vi "n4_betas.vi"(4 "Time":dbl[](array[numeric]), 5 "Tamaño Sn":i32[](array[numeric]), 6 "Analysis":u8, 8 "m":dbl, 9 "P":dbl, 10 "Segmentation A":dbl[](array[numeric]), 11 "Segmentation B":dbl[](array[numeric])) -> (0 "bB":dbl, 1 "X2_tau":dbl[][](array[numeric]), 2 "X2_i":dbl[][](array[numeric]), 3 "bA":dbl)   [LabVIEW 2015]
uses:
  <vilib>/Analysis/baseanly.llb/Mean (DBL).vi
  <vilib>/Analysis/NI_AALBase.lvlib
  <vilib>/Analysis/NI_AALPro.lvlib
panel:
  out "bB_anterior":dbl
  out "bA_anterior":dbl
  out "output array 4":dbl[](array[numeric])
  out "MA 3":dbl
  out "MB 2":dbl
  out "MA 2":dbl
  out "output array 2":dbl[](array[numeric])
  out "MB":dbl
  out "MA":dbl
  out "output array":dbl[](array[numeric])
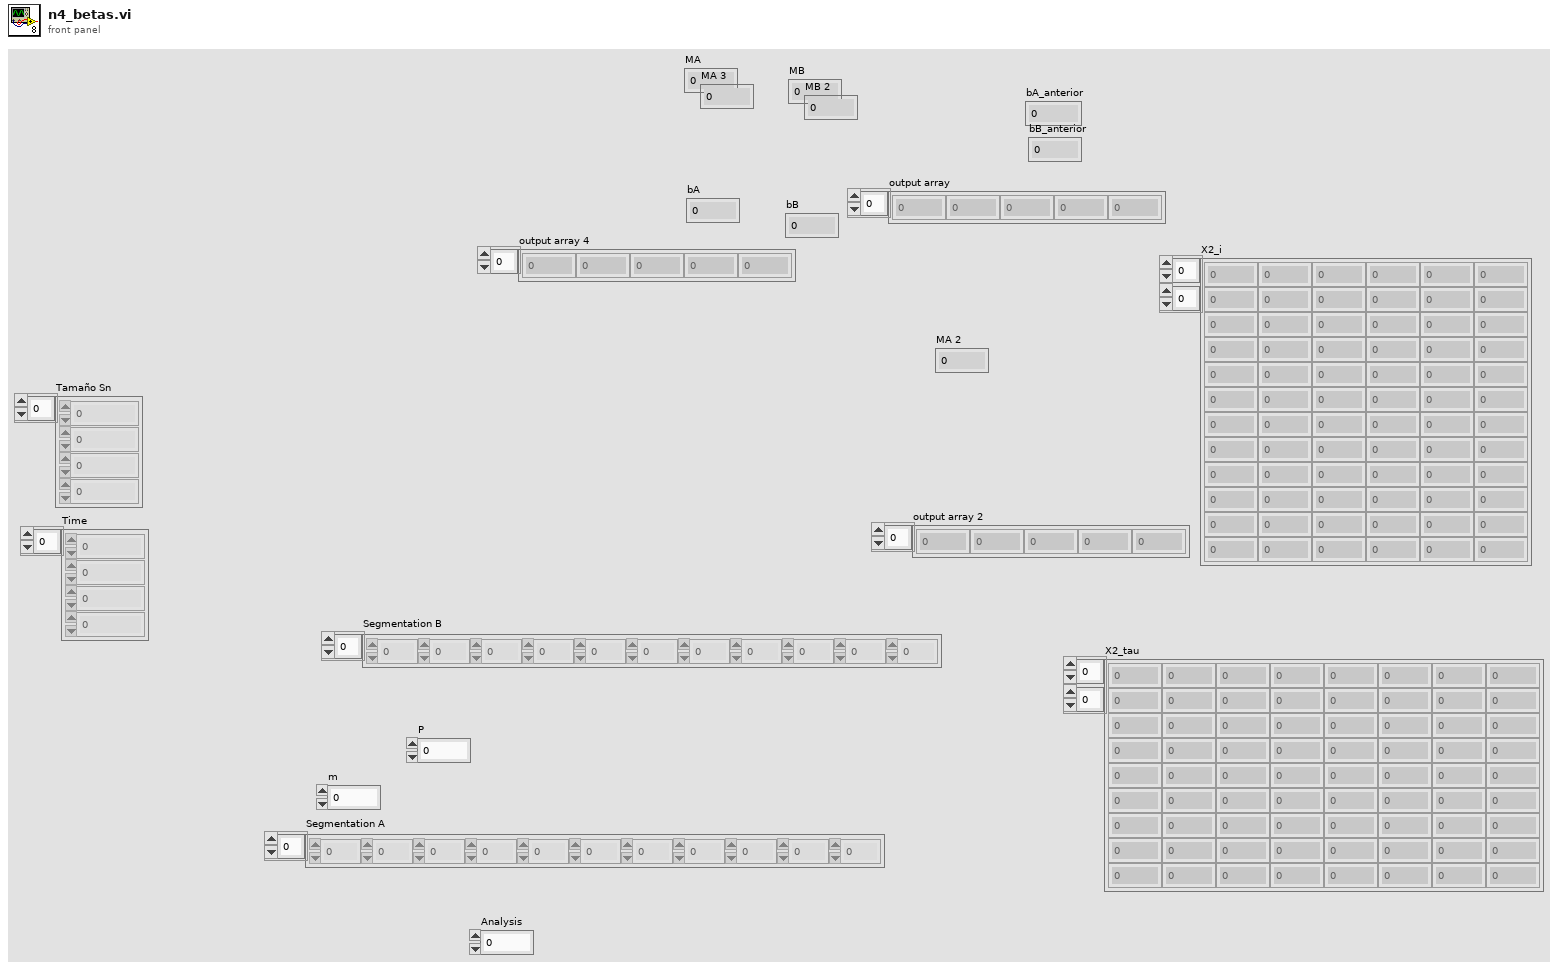
[diagram p1: front panel]
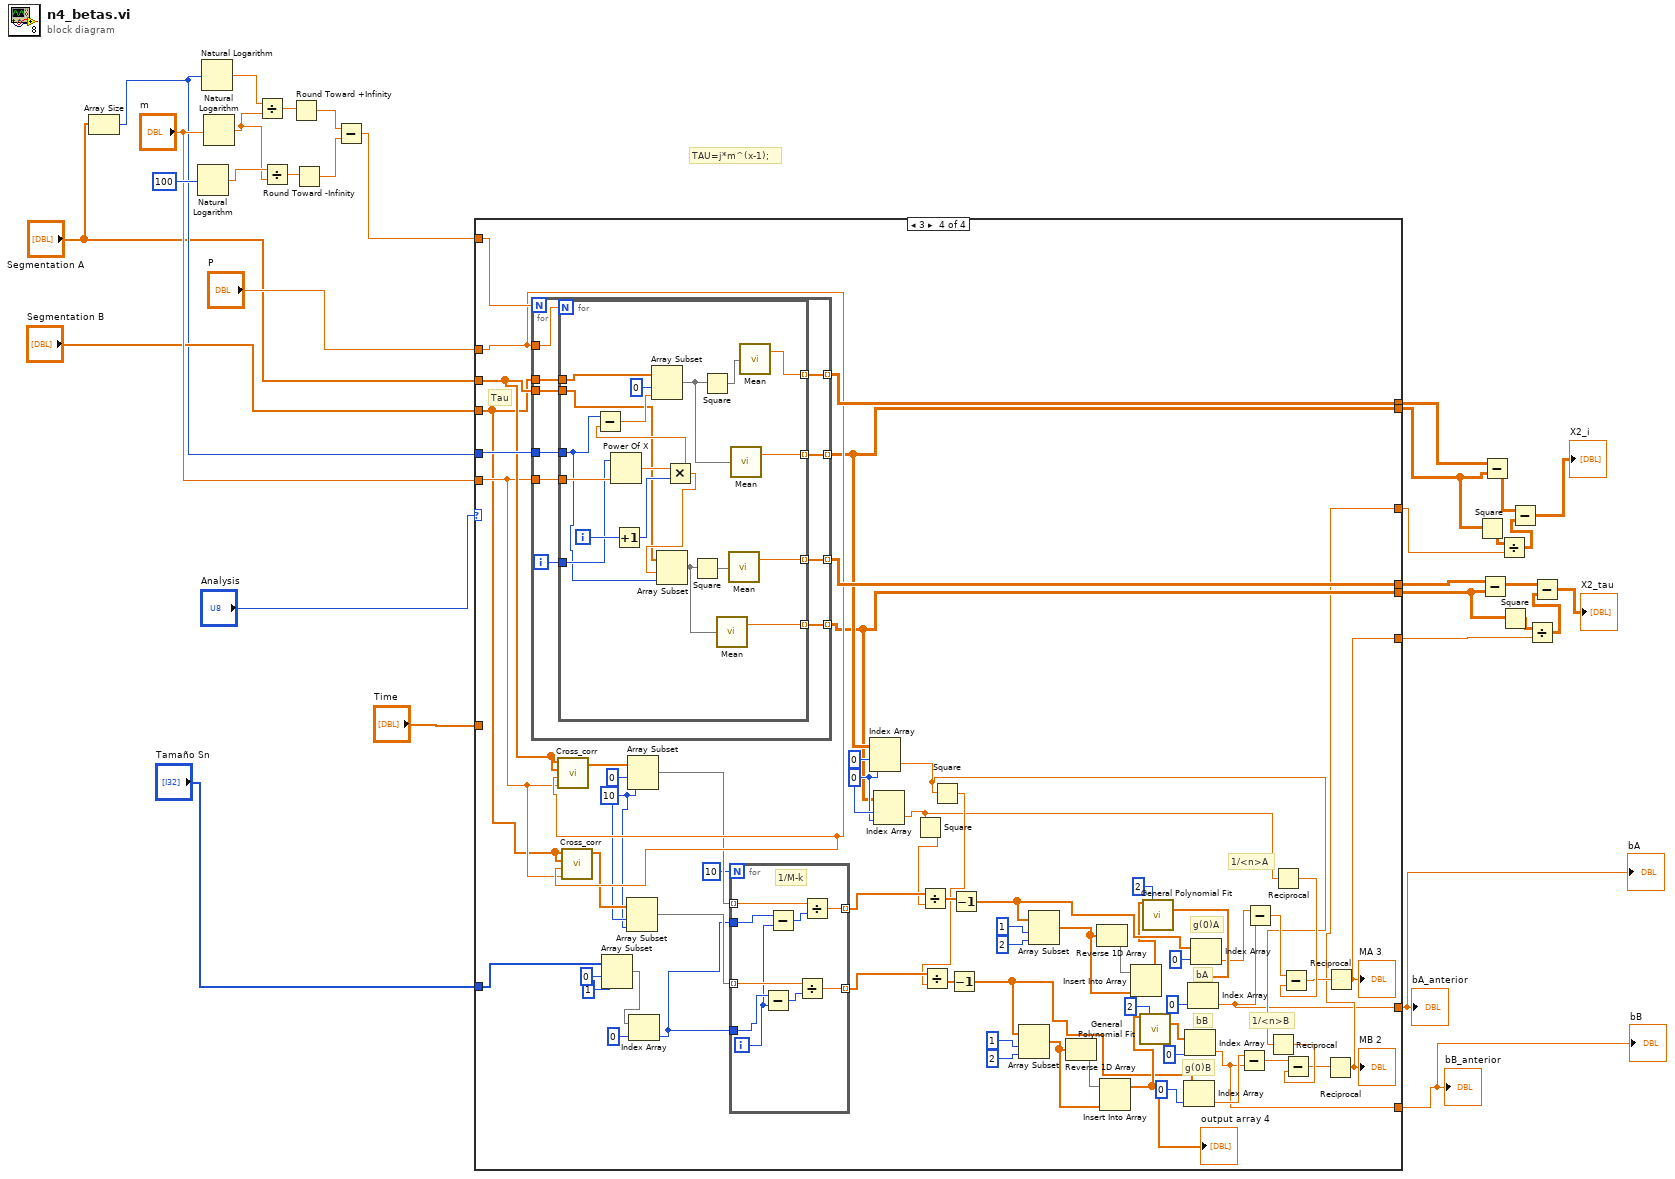
[diagram p0: block diagram]
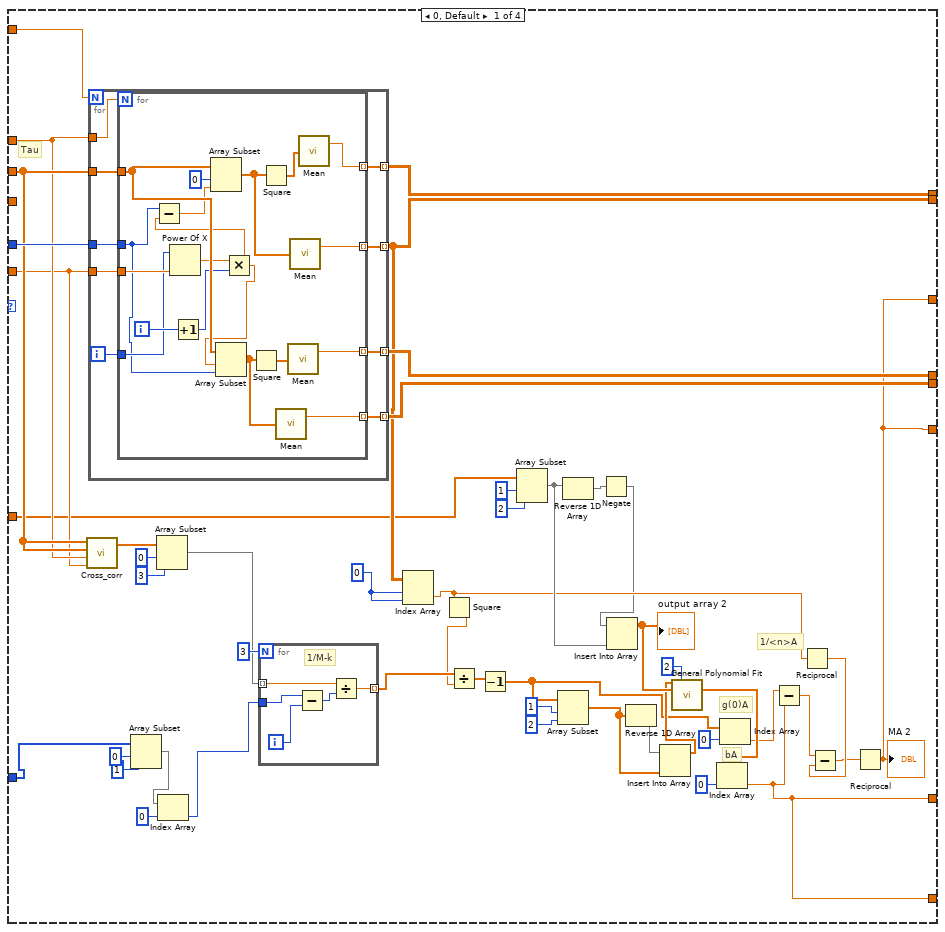
[diagram p2: hidden frame]
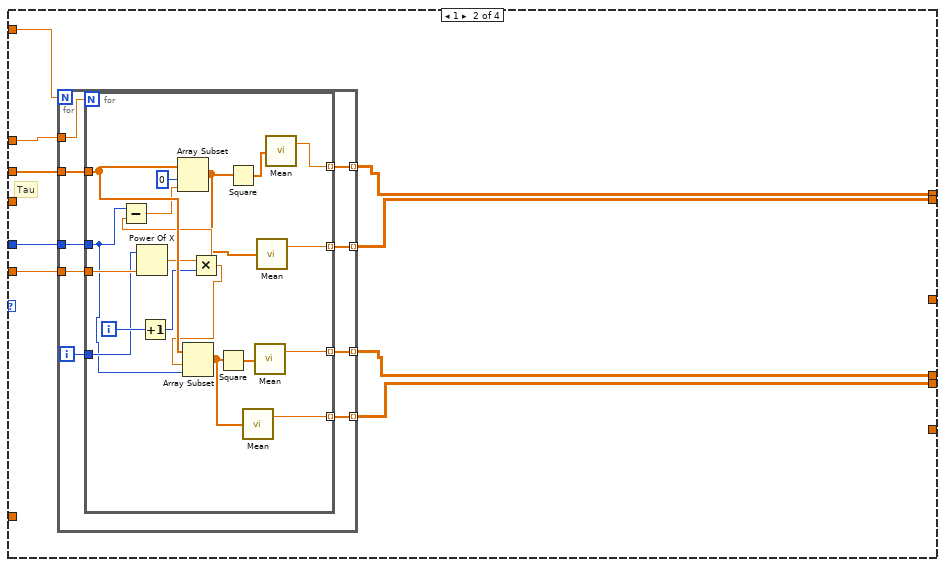
[diagram p3: hidden frame]
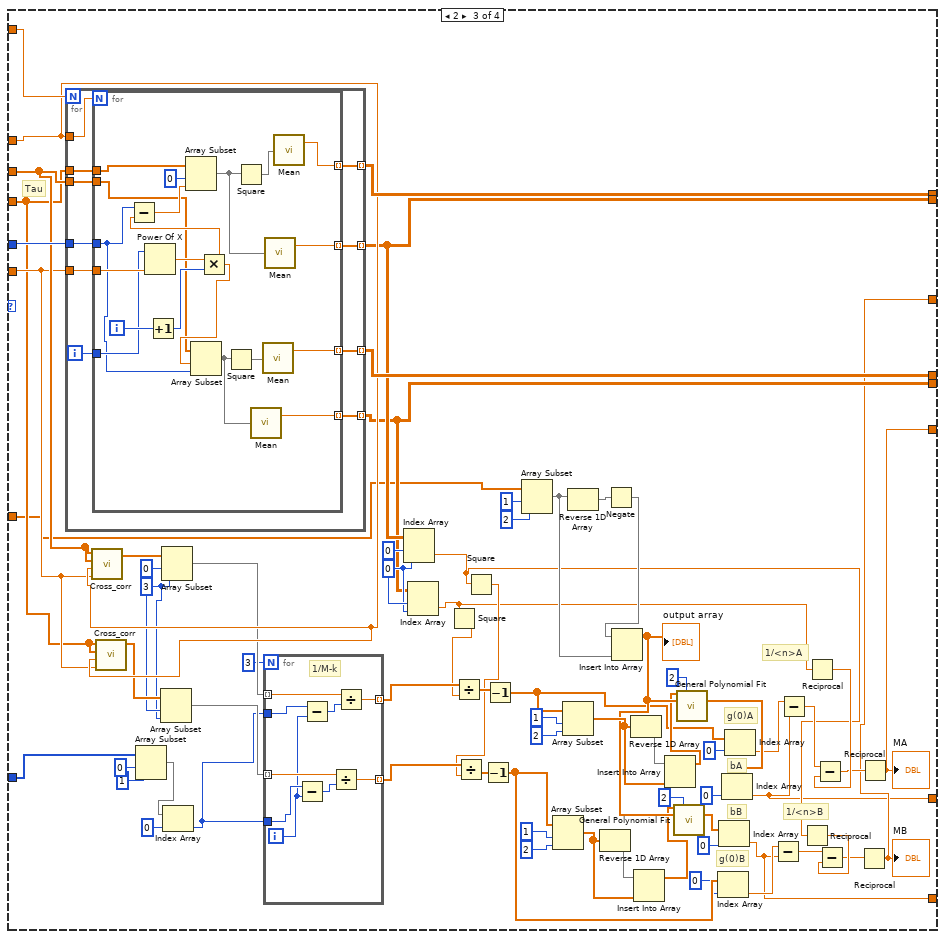
[diagram p4: hidden frame]
diagram:
  # "TAU=j*m^(x-1);"
  n1 = Array Size(array="Segmentation A") -> (size(s)=w18:i32)
  n2 = Natural Logarithm(1:100) -> (0:w30:dbl)
  n3 = Natural Logarithm(1:w18) -> (0:w33:dbl)
  n4 = Natural Logarithm(1:"m") -> (0:w29:dbl)
  n5 = Divide(x=w33, y=w29) -> (x/y=w32:dbl)
  n6 = Divide(x=w30, y=w29) -> (x/y=w27:dbl)
  n7 = Round Toward +Infinity(x=w32) -> (ceil(x): smallest int >= x=w28:dbl)
  n8 = Round Toward -Infinity(1:w27) -> (0:w26:dbl)
  n9 = Subtract(x=w28, y=w26) -> (x-y=w25:dbl)
  n10 = case shown="3" "Analysis" {
    tunnel: "Segmentation A" -> [w45 w122 w217 w320]
    tunnel: w18 -> [w77 w121 w220 w323]
    tunnel: w25 -> [w78 w120 w221 w324]
    tunnel: "m" -> [w43 w119 w215 w318]
    tunnel: "P" -> [w44 w118 w216 w319]
    tunnel: [w81 w117 w219 w322] -> w20
    tunnel: [w40 w116 w202 w305] -> w14
    tunnel: [w80 w115 w218 w321] -> w19
    tunnel: [w79 w114 w177 w288] -> w15
    tunnel: "Segmentation B" -> [_ _ w156 w269]
    tunnel: "Tamaño Sn" -> [w46 _ w208 w311]
    tunnel: [w39 _ w155 w268] -> w12
    tunnel: [w39 _ w154 w267] -> w7
    tunnel: "Time" -> [w35 _ w152 _]
    tunnel: [w34 _ w151 w265] -> w2
    tunnel: [w34 _ w150 w264] -> w1
    frame 0, Default {
      w41 = 0 ("index (col)")
      # "1/<n>A"
      # "bA"
      # "g(0)A"
      # "Tau"
      n11 = call "Cross_corr.vi"("m"=w43, "P"=w44, "input B"=w45, "input A"=w45) -> ("Acc"=w76:dbl[])  [unwired: 5 in, 2 out]
      n12 = for {
        N: w78 -> [_]
        tunnel: w44 -> [w95]
        tunnel: w45 -> [w94]
        tunnel: w77 -> [w93]
        tunnel: w43 -> [w92]
        tunnel: [w91] -> w81 mode=indexing
        tunnel: [w90] -> w40 mode=indexing
        tunnel: [w88] -> w80 mode=indexing
        tunnel: [w87] -> w79 mode=indexing
        i -> [w89]
        n13 = for {
          N: w95 -> [_]
          tunnel: w94 -> [w110]
          tunnel: w93 -> [w102]
          tunnel: w92 -> [w113]
          tunnel: w89 -> [w104]
          tunnel: [w112] -> w91 mode=indexing
          tunnel: [w111] -> w90 mode=indexing
          tunnel: [w108] -> w88 mode=indexing
          tunnel: [w107] -> w87 mode=indexing
          i -> [w106]
          n14 = Power Of X(1:w113, 2:w104) -> (0:w96:dbl)
          n15 = Increment(x=w106) -> (x+1=w105:i32)
          n16 = Multiply(x=w96, y=w105) -> (x*y=w103:dbl)
          n17 = Subtract(x=w102, y=w103) -> (x-y=w100:dbl)
          n18 = Array Subset(array=w110, index=0, length=w100) -> (w101:dbl[])
          n19 = Array Subset(array=w110, index=w103, length=w102) -> (w97:dbl[])
          n20 = Square(x=w97) -> (x^2=w109:dbl[])
          n21 = Square(x=w101) -> (x^2=w98:dbl[])
          n22 = call-poly <vilib>:"Mean.vi"("X"=w97) -> ("mean"=w107:dbl)  [unwired: 1 out]
          n23 = call-poly <vilib>:"Mean.vi"("X"=w109) -> ("mean"=w108:dbl)  [unwired: 1 out]
          n24 = call-poly <vilib>:"Mean.vi"("X"=w101) -> ("mean"=w111:dbl)  [unwired: 1 out]
          n25 = call-poly <vilib>:"Mean.vi"("X"=w98) -> ("mean"=w112:dbl)  [unwired: 1 out]
        }
      }
      n26 = Array Subset(array=w46, index=0, length=1) -> (w71:i32[])
      n27 = Array Subset(array=w76, index=0, length=3) -> (w37:dbl[])
      n28 = Index Array(array=w71, index=0) -> (element=w42:i32)
      n29 = for {
        N: 3 -> [_]
        tunnel: w37 -> [w85] mode=indexing
        tunnel: w42 -> [w84]
        tunnel: [w82] -> w69 mode=indexing
        i -> [w83]
        # "1/M-k"
        n30 = Subtract(x=w84, y=w83) -> (x-y=w86:i32)
        n31 = Divide(x=w85, y=w86) -> (x/y=w82:dbl)
      }
      n32 = Index Array(array=w40, index (row)=w41, index (col)=w41) -> (element=w50:dbl)
      n33 = Square(x=w50) -> (x^2=w56:dbl)
      n34 = Divide(x=w69, y=w56) -> (x/y=w68:dbl[])
      n35 = Decrement(x=w68) -> (x-1=w55:dbl[])
      n36 = Array Subset(array=w35, index=1, length=2) -> (w60:dbl[])
      n37 = Array Subset(array=w55, index=1, length=2) -> (w59:dbl[])
      n38 = Reverse 1D Array(array=w60) -> (reversed array=w65:dbl[])
      n39 = Negate(x=w65) -> (-x=w36:dbl[])
      n40 = Insert Into Array(array=w36, new element=w60) -> (w58:dbl[])  [unwired: 1 in]
      "output array 2" <- w58
      n41 = Reverse 1D Array(array=w59) -> (reversed array=w61:dbl[])
      n42 = Insert Into Array(array=w61, new element=w59) -> (w57:dbl[])  [unwired: 1 in]
      n43 = call <vilib>:"General Polynomial Fit.vi"("Y"=w57, "polynomial order"=2, "X"=w58) -> ("Polynomial Coefficients"=w53:dbl[])  [unwired: 9 in, 3 out]
      n44 = Index Array(array=w53, index=0) -> (element=w34:dbl)
      n45 = Index Array(array=w55, index=0) -> (element=w51:dbl)
      n46 = Subtract(x=w51, y=w34) -> (x-y=w49:dbl)
      n47 = Reciprocal(x=w50) -> (1/x=w48:dbl)
      n48 = Subtract(x=w49, y=w48) -> (x-y=w47:dbl)
      n49 = Reciprocal(x=w47) -> (1/x=w39:dbl)
      "MA 2" <- w39
    }
    frame 1 {
      # "Tau"
      n50 = for {
        N: w120 -> [_]
        tunnel: w118 -> [w131]
        tunnel: w122 -> [w130]
        tunnel: w121 -> [w129]
        tunnel: w119 -> [w128]
        tunnel: [w127] -> w117 mode=indexing
        tunnel: [w126] -> w116 mode=indexing
        tunnel: [w124] -> w115 mode=indexing
        tunnel: [w123] -> w114 mode=indexing
        i -> [w125]
        n51 = for {
          N: w131 -> [_]
          tunnel: w130 -> [w146]
          tunnel: w129 -> [w136]
          tunnel: w128 -> [w149]
          tunnel: w125 -> [w139]
          tunnel: [w148] -> w127 mode=indexing
          tunnel: [w147] -> w126 mode=indexing
          tunnel: [w144] -> w124 mode=indexing
          tunnel: [w142] -> w123 mode=indexing
          i -> [w141]
          n52 = Power Of X(1:w149, 2:w139) -> (0:w138:dbl)
          n53 = Increment(x=w141) -> (x+1=w140:i32)
          n54 = Multiply(x=w138, y=w140) -> (x*y=w137:dbl)
          n55 = Subtract(x=w136, y=w137) -> (x-y=w134:dbl)
          n56 = Array Subset(array=w146, index=0, length=w134) -> (w135:dbl[])
          n57 = Array Subset(array=w146, index=w137, length=w136) -> (w143:dbl[])
          n58 = Square(x=w143) -> (x^2=w145:dbl[])
          n59 = Square(x=w135) -> (x^2=w132:dbl[])
          n60 = call-poly <vilib>:"Mean.vi"("X"=w143) -> ("mean"=w142:dbl)  [unwired: 1 out]
          n61 = call-poly <vilib>:"Mean.vi"("X"=w145) -> ("mean"=w144:dbl)  [unwired: 1 out]
          n62 = call-poly <vilib>:"Mean.vi"("X"=w135) -> ("mean"=w147:dbl)  [unwired: 1 out]
          n63 = call-poly <vilib>:"Mean.vi"("X"=w132) -> ("mean"=w148:dbl)  [unwired: 1 out]
        }
      }
    }
    frame 2 {
      w200 = 0 ("index (col)")
      w201 = 0 ("index (row)")
      w153 = 3 ("length")
      w212 = 0 ("index")
      # "1/<n>B"
      # "1/<n>A"
      # "bB"
      # "bA"
      # "g(0)B"
      # "g(0)A"
      # "Tau"
      n64 = for {
        N: w221 -> [_]
        tunnel: w216 -> [w240]
        tunnel: w156 -> [w239]
        tunnel: w220 -> [w238]
        tunnel: w215 -> [w237]
        tunnel: [w236] -> w219 mode=indexing
        tunnel: [w235] -> w202 mode=indexing
        tunnel: [w233] -> w218 mode=indexing
        tunnel: [w232] -> w177 mode=indexing
        tunnel: w217 -> [w231]
        i -> [w234]
        n65 = for {
          N: w240 -> [_]
          tunnel: w239 -> [w242]
          tunnel: w238 -> [w247]
          tunnel: w237 -> [w259]
          tunnel: w234 -> [w250]
          tunnel: [w258] -> w236 mode=indexing
          tunnel: [w257] -> w235 mode=indexing
          tunnel: [w255] -> w233 mode=indexing
          tunnel: [w253] -> w232 mode=indexing
          tunnel: w231 -> [w241]
          i -> [w252]
          n66 = Power Of X(1:w259, 2:w250) -> (0:w249:dbl)
          n67 = Increment(x=w252) -> (x+1=w251:i32)
          n68 = Multiply(x=w249, y=w251) -> (x*y=w248:dbl)
          n69 = Subtract(x=w247, y=w248) -> (x-y=w245:dbl)
          n70 = Array Subset(array=w242, index=0, length=w245) -> (w246:dbl[])
          n71 = Array Subset(array=w241, index=w248, length=w247) -> (w254:dbl[])
          n72 = Square(x=w254) -> (x^2=w256:dbl[])
          n73 = Square(x=w246) -> (x^2=w243:dbl[])
          n74 = call-poly <vilib>:"Mean.vi"("X"=w254) -> ("mean"=w253:dbl)  [unwired: 1 out]
          n75 = call-poly <vilib>:"Mean.vi"("X"=w256) -> ("mean"=w255:dbl)  [unwired: 1 out]
          n76 = call-poly <vilib>:"Mean.vi"("X"=w246) -> ("mean"=w257:dbl)  [unwired: 1 out]
          n77 = call-poly <vilib>:"Mean.vi"("X"=w243) -> ("mean"=w258:dbl)  [unwired: 1 out]
        }
      }
      n78 = call "Cross_corr.vi"("m"=w215, "P"=w216, "input B"=w217, "input A"=w217) -> ("Acc"=w214:dbl[])  [unwired: 5 in, 2 out]
      n79 = call "Cross_corr.vi"("m"=w215, "P"=w216, "input B"=w156, "input A"=w156) -> ("Acc"=w213:dbl[])  [unwired: 5 in, 2 out]
      n80 = Array Subset(array=w208, index=0, length=1) -> (w205:i32[])
      n81 = Array Subset(array=w213, index=w212, length=w153) -> (w210:dbl[])
      n82 = Array Subset(array=w214, index=w212, length=w153) -> (w211:dbl[])
      n83 = Index Array(array=w205, index=0) -> (element=w203:i32)
      n84 = for {
        N: 3 -> [_]
        tunnel: [w230] -> w198 mode=indexing
        tunnel: w210 -> [w229] mode=indexing
        tunnel: w203 -> [w227]
        tunnel: w211 -> [w225] mode=indexing
        tunnel: w203 -> [w224]
        tunnel: [w222] -> w199 mode=indexing
        i -> [w223]
        # "1/M-k"
        n85 = Subtract(x=w227, y=w223) -> (x-y=w228:i32)
        n86 = Subtract(x=w224, y=w223) -> (x-y=w226:i32)
        n87 = Divide(x=w229, y=w228) -> (x/y=w230:dbl)
        n88 = Divide(x=w225, y=w226) -> (x/y=w222:dbl)
      }
      n89 = Index Array(array=w202, index (row)=w201, index (col)=w200) -> (element=w158:dbl)
      n90 = Index Array(array=w177, index (row)=w201, index (col)=w200) -> (element=w165:dbl)
      n91 = Square(x=w165) -> (x^2=w175:dbl)
      n92 = Divide(x=w199, y=w175) -> (x/y=w197:dbl[])
      n93 = Square(x=w158) -> (x^2=w176:dbl)
      n94 = Divide(x=w198, y=w176) -> (x/y=w196:dbl[])
      n95 = Decrement(x=w196) -> (x-1=w172:dbl[])
      n96 = Decrement(x=w197) -> (x-1=w174:dbl[])
      n97 = Array Subset(array=w152, index=1, length=2) -> (w187:dbl[])
      n98 = Array Subset(array=w172, index=1, length=2) -> (w181:dbl[])
      n99 = Array Subset(array=w174, index=1, length=2) -> (w186:dbl[])
      n100 = Reverse 1D Array(array=w187) -> (reversed array=w193:dbl[])
      n101 = Reverse 1D Array(array=w181) -> (reversed array=w182:dbl[])
      n102 = Negate(x=w193) -> (-x=w192:dbl[])
      n103 = Insert Into Array(array=w192, new element=w187) -> (w180:dbl[])  [unwired: 1 in]
      "output array" <- w180
      n104 = Reverse 1D Array(array=w186) -> (reversed array=w188:dbl[])
      n105 = Insert Into Array(array=w182, new element=w181) -> (w178:dbl[])  [unwired: 1 in]
      n106 = Insert Into Array(array=w188, new element=w186) -> (w179:dbl[])  [unwired: 1 in]
      n107 = call <vilib>:"General Polynomial Fit.vi"("Y"=w178, "polynomial order"=2, "X"=w180) -> ("Polynomial Coefficients"=w168:dbl[])  [unwired: 9 in, 3 out]
      n108 = call <vilib>:"General Polynomial Fit.vi"("Y"=w179, "polynomial order"=2, "X"=w180) -> ("Polynomial Coefficients"=w170:dbl[])  [unwired: 9 in, 3 out]
      n109 = Index Array(array=w172, index=0) -> (element=w157:dbl)
      n110 = Index Array(array=w168, index=0) -> (element=w150:dbl)
      n111 = Index Array(array=w170, index=0) -> (element=w151:dbl)
      n112 = Index Array(array=w174, index=0) -> (element=w166:dbl)
      n113 = Subtract(x=w157, y=w150) -> (x-y=w161:dbl)
      n114 = Subtract(x=w166, y=w151) -> (x-y=w164:dbl)
      n115 = Reciprocal(x=w158) -> (1/x=w162:dbl)
      n116 = Reciprocal(x=w165) -> (1/x=w163:dbl)
      n117 = Subtract(x=w164, y=w163) -> (x-y=w159:dbl)
      n118 = Subtract(x=w161, y=w162) -> (x-y=w160:dbl)
      n119 = Reciprocal(x=w160) -> (1/x=w154:dbl)
      "MB" <- w154
      n120 = Reciprocal(x=w159) -> (1/x=w155:dbl)
      "MA" <- w155
    }
    frame 3 {
      w303 = 0 ("index (col)")
      w304 = 0 ("index (row)")
      w266 = 10 ("length")
      w315 = 0 ("index")
      # "1/<n>B"
      # "1/<n>A"
      # "bB"
      # "bA"
      # "g(0)B"
      # "g(0)A"
      # "Tau"
      n121 = for {
        N: w324 -> [_]
        tunnel: w319 -> [w343]
        tunnel: w269 -> [w342]
        tunnel: w323 -> [w341]
        tunnel: w318 -> [w340]
        tunnel: [w339] -> w322 mode=indexing
        tunnel: [w338] -> w305 mode=indexing
        tunnel: [w336] -> w321 mode=indexing
        tunnel: [w335] -> w288 mode=indexing
        tunnel: w320 -> [w334]
        i -> [w337]
        n122 = for {
          N: w343 -> [_]
          tunnel: w342 -> [w345]
          tunnel: w341 -> [w350]
          tunnel: w340 -> [w362]
          tunnel: w337 -> [w353]
          tunnel: [w361] -> w339 mode=indexing
          tunnel: [w360] -> w338 mode=indexing
          tunnel: [w358] -> w336 mode=indexing
          tunnel: [w356] -> w335 mode=indexing
          tunnel: w334 -> [w344]
          i -> [w355]
          n123 = Power Of X(1:w362, 2:w353) -> (0:w352:dbl)
          n124 = Increment(x=w355) -> (x+1=w354:i32)
          n125 = Multiply(x=w352, y=w354) -> (x*y=w351:dbl)
          n126 = Subtract(x=w350, y=w351) -> (x-y=w348:dbl)
          n127 = Array Subset(array=w345, index=0, length=w348) -> (w349:dbl[])
          n128 = Array Subset(array=w344, index=w351, length=w350) -> (w357:dbl[])
          n129 = Square(x=w357) -> (x^2=w359:dbl[])
          n130 = Square(x=w349) -> (x^2=w346:dbl[])
          n131 = call-poly <vilib>:"Mean.vi"("X"=w357) -> ("mean"=w356:dbl)  [unwired: 1 out]
          n132 = call-poly <vilib>:"Mean.vi"("X"=w359) -> ("mean"=w358:dbl)  [unwired: 1 out]
          n133 = call-poly <vilib>:"Mean.vi"("X"=w349) -> ("mean"=w360:dbl)  [unwired: 1 out]
          n134 = call-poly <vilib>:"Mean.vi"("X"=w346) -> ("mean"=w361:dbl)  [unwired: 1 out]
        }
      }
      n135 = call "Cross_corr.vi"("m"=w318, "P"=w319, "input B"=w320, "input A"=w320) -> ("Acc"=w317:dbl[])  [unwired: 5 in, 2 out]
      n136 = call "Cross_corr.vi"("m"=w318, "P"=w319, "input B"=w269, "input A"=w269) -> ("Acc"=w316:dbl[])  [unwired: 5 in, 2 out]
      n137 = Array Subset(array=w311, index=0, length=1) -> (w308:i32[])
      n138 = Array Subset(array=w316, index=w315, length=w266) -> (w313:dbl[])
      n139 = Array Subset(array=w317, index=w315, length=w266) -> (w314:dbl[])
      n140 = Index Array(array=w308, index=0) -> (element=w306:i32)
      n141 = for {
        N: 10 -> [_]
        tunnel: [w333] -> w301 mode=indexing
        tunnel: w313 -> [w332] mode=indexing
        tunnel: w306 -> [w330]
        tunnel: w314 -> [w328] mode=indexing
        tunnel: w306 -> [w327]
        tunnel: [w325] -> w302 mode=indexing
        i -> [w326]
        # "1/M-k"
        n142 = Subtract(x=w330, y=w326) -> (x-y=w331:i32)
        n143 = Subtract(x=w327, y=w326) -> (x-y=w329:i32)
        n144 = Divide(x=w332, y=w331) -> (x/y=w333:dbl)
        n145 = Divide(x=w328, y=w329) -> (x/y=w325:dbl)
      }
      n146 = Index Array(array=w305, index (row)=w304, index (col)=w303) -> (element=w271:dbl)
      n147 = Index Array(array=w288, index (row)=w304, index (col)=w303) -> (element=w278:dbl)
      n148 = Square(x=w278) -> (x^2=w286:dbl)
      n149 = Divide(x=w302, y=w286) -> (x/y=w300:dbl[])
      n150 = Square(x=w271) -> (x^2=w287:dbl)
      n151 = Divide(x=w301, y=w287) -> (x/y=w299:dbl[])
      n152 = Decrement(x=w299) -> (x-1=w260:dbl[])
      n153 = Decrement(x=w300) -> (x-1=w262:dbl[])
      n154 = Array Subset(array=w260, index=1, length=2) -> (w289:dbl[])
      n155 = Array Subset(array=w262, index=1, length=2) -> (w294:dbl[])
      n156 = Reverse 1D Array(array=w289) -> (reversed array=w290:dbl[])
      n157 = Reverse 1D Array(array=w294) -> (reversed array=w295:dbl[])
      n158 = Insert Into Array(array=w290, new element=w289) -> (w263:dbl[])  [unwired: 1 in]
      "output array 4" <- w263
      n159 = Insert Into Array(array=w295, new element=w294) -> (w261:dbl[])  [unwired: 1 in]
      n160 = call <vilib>:"General Polynomial Fit.vi"("Y"=w263, "polynomial order"=2) -> ("Polynomial Coefficients"=w281:dbl[])  [unwired: 10 in, 3 out]
      n161 = call <vilib>:"General Polynomial Fit.vi"("Y"=w261, "polynomial order"=2) -> ("Polynomial Coefficients"=w283:dbl[])  [unwired: 10 in, 3 out]
      n162 = Index Array(array=w260, index=0) -> (element=w270:dbl)
      n163 = Index Array(array=w281, index=0) -> (element=w264:dbl)
      n164 = Index Array(array=w283, index=0) -> (element=w265:dbl)
      n165 = Index Array(array=w262, index=0) -> (element=w279:dbl)
      n166 = Subtract(x=w270, y=w264) -> (x-y=w274:dbl)
      n167 = Subtract(x=w279, y=w265) -> (x-y=w277:dbl)
      n168 = Reciprocal(x=w271) -> (1/x=w275:dbl)
      n169 = Reciprocal(x=w278) -> (1/x=w276:dbl)
      n170 = Subtract(x=w277, y=w276) -> (x-y=w272:dbl)
      n171 = Subtract(x=w274, y=w275) -> (x-y=w273:dbl)
      n172 = Reciprocal(x=w273) -> (1/x=w267:dbl)
      "MB 2" <- w267
      n173 = Reciprocal(x=w272) -> (1/x=w268:dbl)
      "MA 3" <- w268
    }
  }
  "bA" <- w2
  "bB" <- w1
  "bA_anterior" <- w2
  "bB_anterior" <- w1
  n174 = Square(x=w14) -> (x^2=w6:dbl[][])
  n175 = Subtract(x=w19, y=w15) -> (x-y=w9:dbl[][])
  n176 = Subtract(x=w20, y=w14) -> (x-y=w13:dbl[][])
  n177 = Divide(x=w6, y=w7) -> (x/y=w5:dbl[][])
  n178 = Square(x=w15) -> (x^2=w11:dbl[][])
  n179 = Subtract(x=w13, y=w5) -> (x-y=→"X2_i":dbl[][])
  n180 = Divide(x=w11, y=w12) -> (x/y=w10:dbl[][])
  n181 = Subtract(x=w9, y=w10) -> (x-y=→"X2_tau":dbl[][])
